vi "Get Unique Name.vi"(9 "error in":errorcluster, 10 "Name":string, 11 "Branch":refnum<data-value>) -> (1 "error out":errorcluster, 2 "Unique Name":string, 3 "Branch":refnum<data-value>)   [LabVIEW 2019, in "Tree.lvclass"]
uses:
  Tree.lvclass
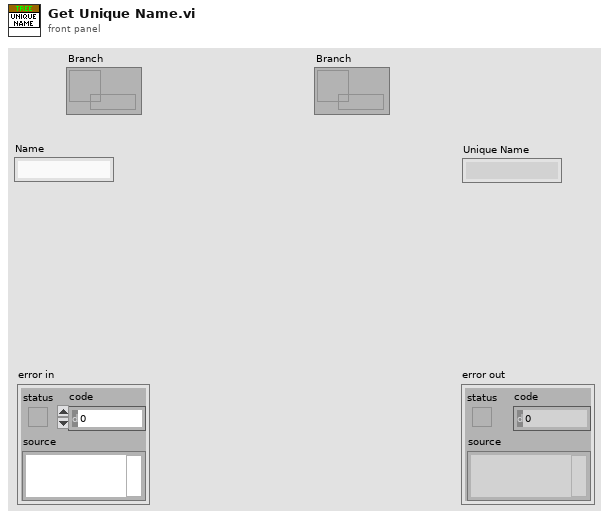
[diagram p1: front panel]
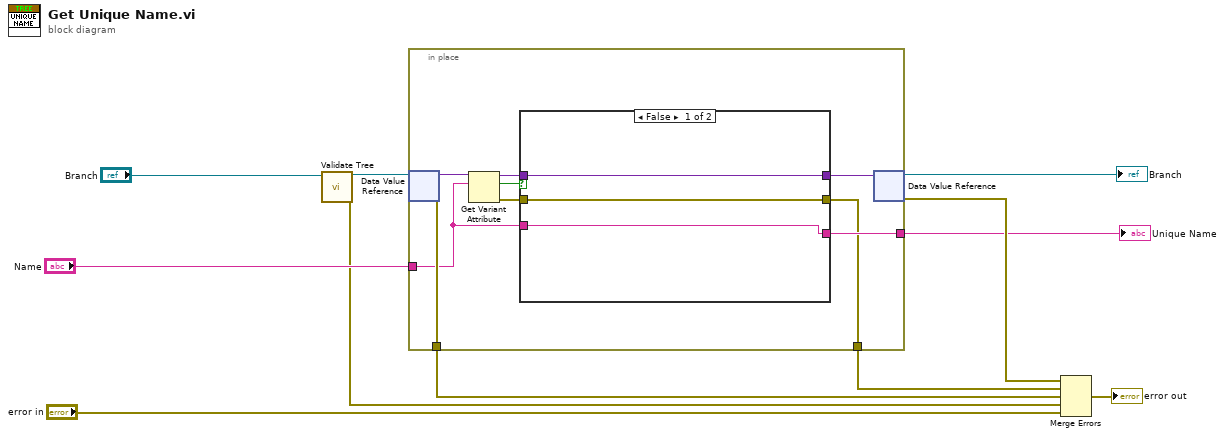
[diagram p0: block diagram]
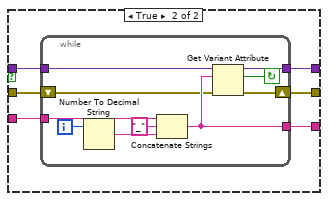
[diagram p2: hidden frame]
diagram:
  n1 = call "Validate Tree.vi"("Branch Reference In"="Branch") -> ("error out"=w1:errorcluster, "Branch Reference Out"=w3:refnum<data-value>)  [unwired: 9 in]
  n2 = in-place {
    in-place-border: [w20] -> w8
    in-place-border: "Name" -> [w15]
    in-place-border: [w16] -> w6
    in-place-border: [w12] -> w5
    n3 = in-place-dvr #1(w3) -> (w19:variant, w20:errorcluster)
    n4 = Get Variant Attribute(Variant=w19, name=w15) -> (duplicate Variant=w18:variant, found=w14:bool, error out=w13:errorcluster)  [unwired: 2 in, 1 out]
    n5 = case shown="False" w14 {
      tunnel: [w22 w29] -> w16
      tunnel: [w23 w28] -> w17
      tunnel: w18 -> [w23 w27]
      tunnel: w15 -> [w22 w26]
      tunnel: w13 -> [w21 w25]
      tunnel: [w21 w24] -> w12
      frame False {
      }
      frame True {
        n6 = while {
          tunnel: w27 -> [w35]
          tunnel: w26 -> [w37]
          tunnel: [w33] -> w29
          tunnel: [w32] -> w28
          shift-right: [w31] -> w24
          shift-left: w25 -> [w30]
          i -> [w39]
          stop <- w34 continue-if-true
          n7 = Number To Decimal String(number=w39) -> (decimal integer string=w36:string)  [unwired: 1 in]
          n8 = Concatenate Strings(w37, "_" ("string"), w36) -> (w33:string)
          n9 = Get Variant Attribute(Variant=w35, name=w33, error in=w30) -> (duplicate Variant=w32:variant, found=w34:bool, error out=w31:errorcluster)  [unwired: 1 in, 1 out]
        }
      }
    }
    n10 = in-place-dvr #1(w17) -> (→"Branch":refnum<data-value>, w9:errorcluster)
  }
  "Unique Name" <- w6
  n11 = Merge Errors(w9, w5, w8, w1, "error in") -> (→"error out":errorcluster)
